vi "Draw_Cage_circle_chord_segment.vi"(0 "Picture refnum in":T2, 5 "Bounding rectangle in":T1, 7 "Fill color":u32(colorbox)=13816530, 9 "Outline color":u32(colorbox), 11 "Error In":errorcluster, 12 "Border thickness, pix":i32=6, 13 "Cage floor color":u32(colorbox)=9868950) -> (4 "Picture refnum out":T2, 6 "Bounding rectangle out":T1, 15 "Error Out":errorcluster)   [LabVIEW 2018, in "Cage Diagram.lvlib"]
uses:
  Cage Diagram.lvlib
  <vilib>/vision/Image Controls.llb/IMAQ Image.ctl
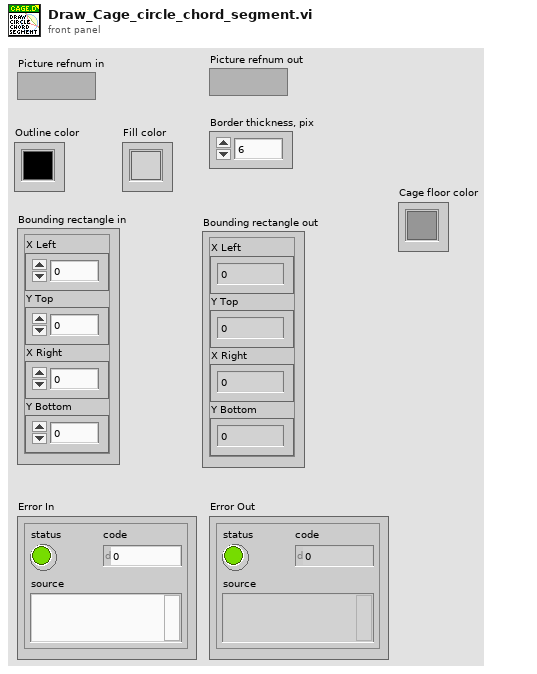
[diagram p1: front panel]
types:
  T1 = cluster{"X Left":dbl, "Y Top":dbl, "X Right":dbl, "Y Bottom":dbl}
  T2 = typedef "IMAQ Image.ctl" = refnum<image>
  T3 = cluster{"X Left":dbl, "Y Top":dbl, "X Right":dbl, dbl}
  T4 = cluster{"X Left":dbl, dbl, "X Right":dbl, "Y Bottom":dbl}
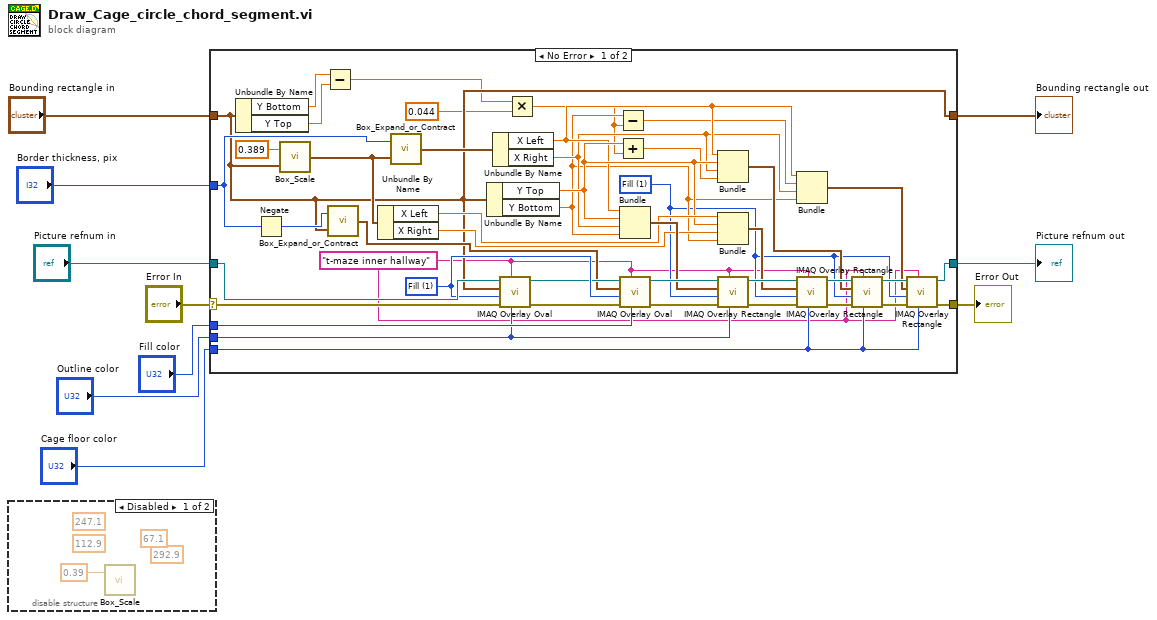
[diagram p0: block diagram]
diagram:
  n1 = disable-structure shown="Disabled" {
    frame Disabled {
      (unwired) 292.9 ("End Angle (degrees)")
      (unwired) 67.1 ("Start Angle (degrees)")
      (unwired) 247.1 ("End Angle (degrees)")
      (unwired) 112.9 ("Start Angle (degrees)")
      n2 = call "Box_Scale.vi"("Scale factor"=0.39) -> ()  [unwired: 1 in, 1 out]
    }
    frame Enabled {
    }
  }
  n3 = case shown="No Error" "Error In" {
    selector: "Error In" -> [w55 w58]
    tunnel: [w23 w58] -> w9
    tunnel: "Outline color" -> [w45 _]
    tunnel: [w21 w57] -> w7
    tunnel: "Picture refnum in" -> [w54 w57]
    tunnel: "Fill color" -> [w50 _]
    tunnel: "Bounding rectangle in" -> [w29 w56]
    tunnel: [w29 w56] -> w3
    tunnel: "Border thickness, pix" -> [w40 _]
    tunnel: "Cage floor color" -> [w14 _]
    frame No Error {
      w12 = "t-maze inner hallway" ("Group")
      w13 = u32 1 items=["Frame", "Fill"] ("Drawing Mode (Frame)")
      w53 = u32 1 items=["Frame", "Fill"] ("Drawing Mode (Frame)")
      n4 = Unbundle By Name(w29) -> ("Y Bottom"=w28:dbl, "Y Top"=w27:dbl)
      n5 = Negate(x=w40) -> (-x=w41:i32)
      n6 = call "Box_Scale.vi"("Rectangle in"=w29, "Scale factor"=0.389) -> ("Rectangle out"=w39:T1)
      n7 = Subtract(x=w28, y=w27) -> (x-y=w26:dbl)
      n8 = call "Box_Expand_or_Contract.vi"("Rectangle in"=w29, "Expand/Contract"=w41) -> ("Rectangle out"=w49:T1)
      n9 = Unbundle By Name(w39) -> ("X Left"=w42:dbl, "X Right"=w43:dbl)
      n10 = call "Box_Expand_or_Contract.vi"("Rectangle in"=w39, "Expand/Contract"=w40) -> ("Rectangle out"=w35:T1)
      n11 = Unbundle By Name(w29) -> ("Y Top"=w31:dbl, "Y Bottom"=w18:dbl)
      n12 = Unbundle By Name(w35) -> ("X Left"=w20:dbl, "X Right"=w19:dbl)
      n13 = call "IMAQ Overlay Oval"("Color"=w45, "Group"=w12, "error in (no error)"=w55, "Drawing Mode (Frame)"=w53, "Bounding Rectangle"=w29, "Image"=w54) -> ("error out"=w51:errorcluster, "Image Out"=w52:T2)  [unwired: 4 in]
      n14 = Multiply(x=w26, y=0.044) -> (x*y=w17:dbl)
      n15 = Subtract(x=w18, y=w17) -> (x-y=w16:dbl)
      n16 = Add(x=w31, y=w17) -> (x+y=w30:dbl)
      n17 = Bundle("X Left"=w20, "Y Top"=w31, "X Right"=w19, "Y Bottom"=w18) -> (w44:T1)  [unwired: 1 in]
      n18 = call "IMAQ Overlay Oval"("Color"=w50, "Group"=w12, "error in (no error)"=w51, "Drawing Mode (Frame)"=w53, "Bounding Rectangle"=w49, "Image"=w52) -> ("error out"=w46:errorcluster, "Image Out"=w47:T2)  [unwired: 4 in]
      n19 = Bundle("X Left"=w20, "Y Top"=w31, "X Right"=w19, w30) -> (w32:T3)  [unwired: 1 in]
      n20 = Bundle("X Left"=w42, "Y Top"=w31, "X Right"=w43, "Y Bottom"=w18) -> (w36:T1)  [unwired: 1 in]
      n21 = call "IMAQ Overlay Rectangle"("Color"=w45, "Group"=w12, "error in (no error)"=w46, "Drawing Mode (Frame)"=w13, "Rectangle"=w44, "Image"=w47) -> ("error out"=w37:errorcluster, "Image Out"=w38:T2)  [unwired: 4 in]
      n22 = Bundle("X Left"=w20, w16, "X Right"=w19, "Y Bottom"=w18) -> (w15:T4)  [unwired: 1 in]
      n23 = call "IMAQ Overlay Rectangle"("Color"=w14, "Group"=w12, "error in (no error)"=w37, "Drawing Mode (Frame)"=w13, "Rectangle"=w36, "Image"=w38) -> ("error out"=w33:errorcluster, "Image Out"=w34:T2)  [unwired: 4 in]
      n24 = call "IMAQ Overlay Rectangle"("Color"=w14, "Group"=w12, "error in (no error)"=w33, "Drawing Mode (Frame)"=w13, "Rectangle"=w32, "Image"=w34) -> ("error out"=w24:errorcluster, "Image Out"=w22:T2)  [unwired: 4 in]
      n25 = call "IMAQ Overlay Rectangle"("Color"=w14, "Group"=w12, "error in (no error)"=w24, "Drawing Mode (Frame)"=w13, "Rectangle"=w15, "Image"=w22) -> ("error out"=w23:errorcluster, "Image Out"=w21:T2)  [unwired: 4 in]
    }
    frame Error {
    }
  }
  "Error Out" <- w9
  "Picture refnum out" <- w7
  "Bounding rectangle out" <- w3
